vi "FRC Particle Classification Example.vi"() -> (1 "Highest Avg Score":dbl)   [LabVIEW 2015]
uses:
  <vilib>/Rock Robotics/WPI/Camera/WPI_CameraSettings Read MJPG.ctl
  <vilib>/Rock Robotics/WPI/Camera/WPI_CameraImageSize.ctl
  D:/LabView 2015/examples/FRC/roboRIO/Vision/2016 Vision Example/Vision Support Code/Camera Types.ctl
  <vilib>/vision/NI_Vision_Development_Module.lvlib
panel:
  in  "Std Devs for Calibration":cluster{"H":dbl, "S":dbl, "V":dbl}={"H"=4.0, "S"=6.0, "V"=6.0}
  in  "Min Score Threshold":i32=70
  in  "Camera Type":T1=enum."MS HD3000 square"
  in  "image files":string[](array[string])
  out "Detected Targets":T2(array[cluster]) {"Normalized Rect"."Numeric 5" format="%#_2g"; "Normalized Rect"."Numeric 3" format="%#_2g"; "Normalized Rect"."Numeric 2" format="%#_2g"; "Normalized Rect"."Numeric" format="%#_2g"}
  in  "Annotation Limit":dbl=75.0
  in  "Source":enum32{"Files", "Camera"}(tab)
  in  "Images":i32(listbox)
  in  "Folder Location":path=path "C:/Program Files (x86)/National Instruments/LabVIEW 2015/examples/FRC/roboRIO/Vision/2016 Vision Example/Sample Images/Real Tower"
  in  "Camera Settings":T3={"fps"=20, "compression"=30, "Image Size"=enum."320x240"}
  in  "Camera Address":string="USB 1"
  in  "Annotate":bool=TRUE
  out "Sorted Scores":T5(array[cluster]) {"?" format="%#_3g"; "Class Score" format="%#_3g"}
  out "Qualified Particles":i32
  in  "LED Color":T6={"Hue"={110.68604567358754, 149.18771039657545}, "Sat"={35.35714285714287, 255.0}, "Val"={91.0, 255.0}} {"Hue" scale=0.0..255.0 scale format="%#_3g"}
  out "Masked":T7(plugin-control)
  out "Original Image":T7(plugin-control)
  # "Instructions:\nUse Source to select image files from a directory, or use a USB or IP camera connected to your laptop.\nUse LED Color to threshold and build particles. Adjust HSV values to improve masking.\nClick and draw a line in Original Image to auto-calibrate to the LED color. You may need to widen Sat and Val.\nAnnotations draw a rectangle around \"good\" particles with scores from top to bottom."
  # "ID Score"
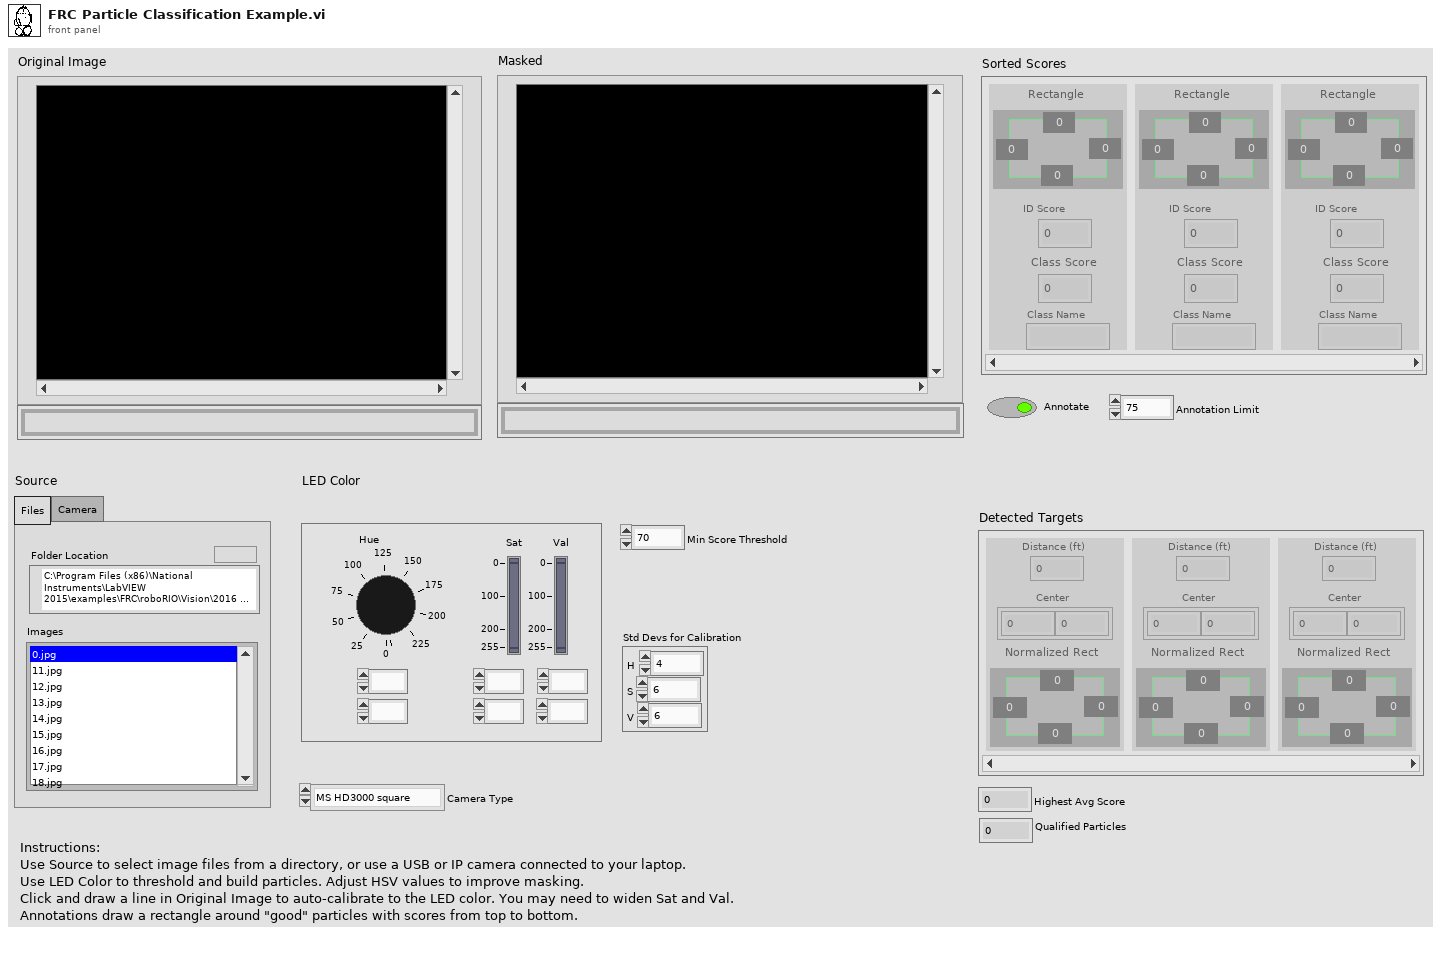
[diagram p1: front panel]
types:
  T1 = typedef "Camera Types.ctl" = enum16{"206", "1011", "1013", "MS HD3000 square", "MS HD3000 640x480"}
  T2 = cluster{"Distance (ft)":dbl, "Center":cluster{dbl, dbl}, "Normalized Rect":cluster{"Numeric":dbl, "Numeric 2":dbl, "Numeric 3":dbl, "Numeric 5":dbl}}[]
  T3 = typedef "WPI_CameraSettings Read MJPG.ctl" = cluster{"fps":i32, "compression":i32, "Image Size":T4}
  T4 = typedef "WPI_CameraImageSize.ctl" = enum16{"640x480", "320x240", "160x120", "Custom"}
  T5 = cluster{"Rectangle":cluster{"Numeric":dbl, "Numeric 2":dbl, "Numeric 3":dbl, "Numeric 5":dbl}, dbl, "Class Score":dbl, "Class Name":string}[]
  T6 = cluster{"Hue":cluster{dbl, dbl}, "Sat":cluster{dbl, dbl}, "Val":cluster{dbl, dbl}}
  T7 = typedef "IMAQ Image.ctl" = refnum<image>
  T8 = typedef "Particle Parameters" = i32
  T9 = typedef "Image Type" = u32
  T10 = typedef "IMAQ Classifier Session.ctl" = refnum<k1>
  T11 = cluster{"Numeric":dbl, "Numeric":dbl, "Numeric":dbl, "Numeric":dbl, dbl}
  T12 = cluster{cluster{dbl, dbl}, cluster{dbl, dbl}, cluster{dbl, dbl}}
  T13 = typedef "ROI Descriptor" = cluster{"Global Rectangle":i32[], "Contours":cluster{"ID":enum32{"External", "Internal"}, "Type":u32, "Coordinates":i32[]}[]}
  T14 = cluster{"Classification Score":sgl, "Identification Score":sgl}
  T15 = cluster{"Classification Score":dbl, "Identification Score":dbl}
  T16 = cluster{"Numeric":dbl, "Numeric":dbl, "Numeric":dbl, "Numeric":dbl}
  T17 = cluster{cluster{"Numeric":dbl, "Numeric":dbl, "Numeric":dbl, "Numeric":dbl}, "Identification Score":dbl, "Classification Score":dbl, "Class":string}
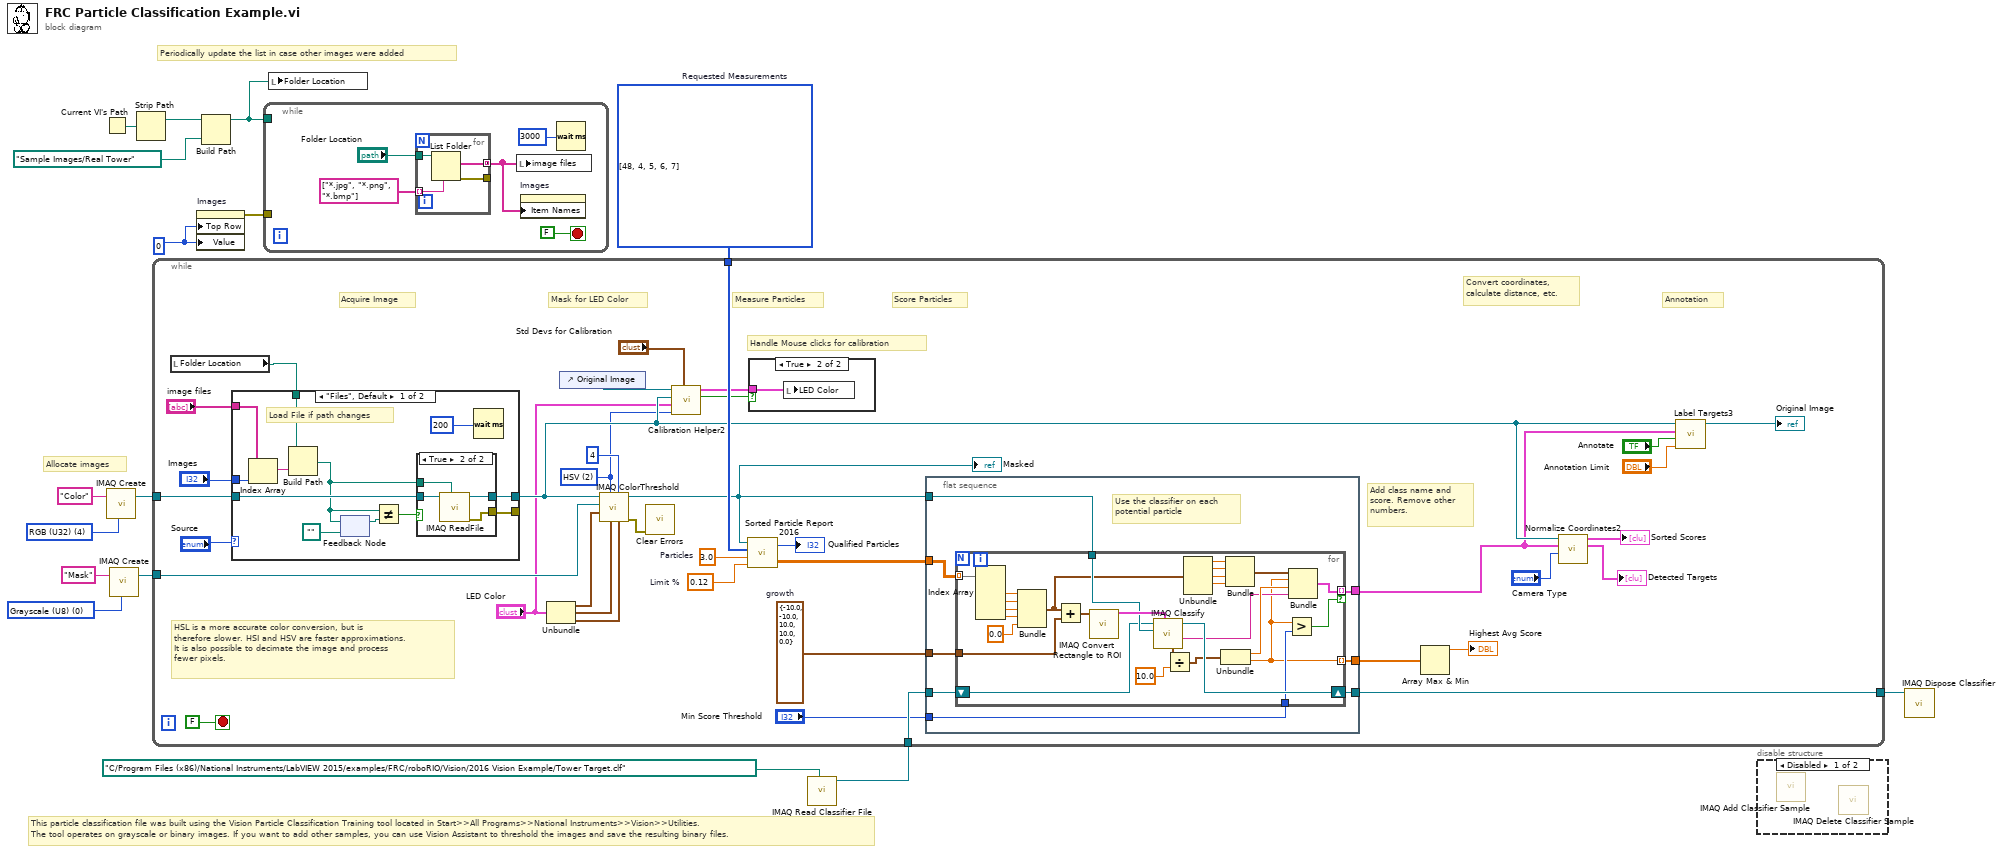
[diagram p0: block diagram]
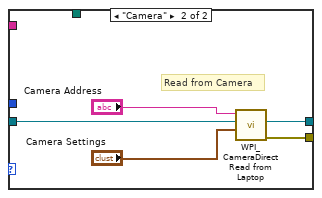
[diagram p5: hidden frame]
diagram:
  w3 = u32 0 ("milliseconds to wait")
  w10 = T8[] [48, 4, 5, 6, 7] items=["Center of Mass X", "Center of Mass Y", "First Pixel X", "First Pixel Y", "Bounding Rect Left", "Bounding Rect Top", "Bounding Rect Right", "Bounding Rect Bottom", "Max Feret Diameter Start X", "Max Feret Diameter Start Y", "Max Feret Diameter End X", "Max Feret Diameter End Y", "Max Horiz. Segment Length Left", "Max Horiz. Segment Length Right", "Max Horiz. Segment Length Row", "-", "Bounding Rect Width", "Bounding Rect Height", "Bounding Rect Diagonal", "Perimeter", "Convex Hull Perimeter", "Holes' Perimeter", "Max Feret Diameter", "Equivalent Ellipse Major Axis", "Equivalent Ellipse Minor Axis", "Equivalent Ellipse Minor Axis (Feret)", "Equivalent Rect Long Side", "Equivalent Rect Short Side", "Equivalent Rect Diagonal", "Equivalent Rect Short Side (Feret)", "Average Horiz. Segment Length", "Average Vert. Segment Length", "Hydraulic Radius", "Waddel Disk Diameter", "-", "Area", "Holes' Area", "Particle & Holes' Area", "Convex Hull Area", "Image Area", "-", "Number of Holes", "Number of Horiz. Segments", "Number of Vert. Segments", "-", "Orientation", "Max Feret Diameter Orientation", "-", "% Area/Image Area", "% Area/(Particle & Holes' Area)", "Ratio of Equivalent Ellipse Axes", "Ratio of Equivalent Rect Sides", "-", "Elongation Factor", "Compactness Factor", "Heywood Circularity Factor", "Type Factor", "-", "Sum X", "Sum Y", "Sum XX", "Sum XY", "Sum YY", "Sum XXX", "Sum XXY", "Sum XYY", "Sum YYY", "-", "Moment of Inertia XX", "Moment of Inertia XY", "Moment of Inertia YY", "Moment of Inertia XXX", "Moment of Inertia XXY", "Moment of Inertia XYY", "Moment of Inertia YYY", "Norm. Moment of Inertia XX", "Norm. Moment of Inertia XY", "Norm. Moment of Inertia YY", "Norm. Moment of Inertia XXX", "Norm. Moment of Inertia XXY", "Norm. Moment of Inertia XYY", "Norm. Moment of Inertia YYY", "Hu Moment 1", "Hu Moment 2", "Hu Moment 3", "Hu Moment 4", "Hu Moment 5", "Hu Moment 6", "Hu Moment 7"]  # Requested Measurements
  w13 = T9 0 items=["Grayscale (U8)", "Grayscale (I16)", "Grayscale (SGL)", "Complex (CSG)", "RGB (U32)", "HSL (U32)", "RGB (U64)", "Grayscale (U16)"] ("Image Type")
  w15 = T9 4 items=["Grayscale (U8)", "Grayscale (I16)", "Grayscale (SGL)", "Complex (CSG)", "RGB (U32)", "HSL (U32)", "RGB (U64)", "Grayscale (U16)"] ("Image Type")
  # "This particle classification file was built using the Vision Particle Classification Training tool located in Start>>All Programs>>National Instruments>>Vision>>Utilities.\nThe tool operates on grayscale or binary images. If you want to add other samples, you can use Vision Assistant to threshold the images and save the resulting binary files."
  # "Periodically update the list in case other images were added"
  # "Allocate images"
  n1 = Current VI's Path() -> (path=w9:path)
  n2 = call "IMAQ Create"("Image Name"="Color", "Image Type"=w15) -> ("New Image"=w14:T7)  [unwired: 2 in, 2 out]
  n3 = call "IMAQ Create"("Image Name"="Mask", "Image Type"=w13) -> ("New Image"=w11:T7)  [unwired: 2 in, 2 out]
  n4 = Strip Path(path=w9) -> (stripped path=w4:path)  [unwired: 1 out]
  n5 = property on="Images" class="LstBox (strict)"("Top Row"=w3, "Value"=w3) -> (error out=w2:errorcluster)  [unwired: 2 in, 1 out]
  n6 = Build Path(base path=w4, name or relative path=path "Sample Images/Real Tower" ("Folder Location")) -> (appended path=w1:path)
  n7 = while {
    tunnel: w1 -> [_]
    tunnel: w2 -> [_]
    stop <- FALSE stop-if-true
    n8 = for {
      tunnel: [w25] -> w19 mode=concatenating
      tunnel: "Folder Location" -> [w24]
      tunnel: [w23] -> _
      tunnel: string[] ["*.jpg", "*.png", "*.bmp"] -> [w22] mode=indexing
      n9 = List Folder(path=w24, pattern=w22) -> (filenames=w25:string[], error out=w23:errorcluster)  [unwired: 2 in, 2 out]
    }
    n10 = local write "image files"(w19) -> ()
    n11 = property on="Images" class="LstBox (strict)"("Item Names"=w19) -> ()  [unwired: 2 in, 2 out]
    n12 = Wait (ms)(milliseconds to wait=u32 3000) -> ()  [unwired: 1 out]
  }
  n13 = local write "Folder Location"(w1) -> ()
  n14 = call "IMAQ Read Classifier File"("File Path"=path "C:/Program Files (x86)/National Instruments/LabVIEW 2015/examples/FRC/roboRIO/Vision/2016 Vision Example/Tower Target.clf" ("appended path")) -> ("Classifier Session"=w7:T10)  [unwired: 3 in, 7 out]
  n15 = while {
    tunnel: w14 -> [w62]
    tunnel: w11 -> [w60]
    tunnel: w10 -> [w56]
    tunnel: w7 -> [w38]
    tunnel: [w35] -> w6
    stop <- FALSE stop-if-true
    w39 = T11 {"Numeric"=-10.0, "Numeric"=-10.0, "Numeric"=10.0, "Numeric"=10.0, 0.0}  # growth
    w53 = 0.12  # Limit %
    w55 = 3.0  # Particles
    w43 = u16 2 items=["RGB", "HSL", "HSV", "HSI"] ("Color Mode")
    # "Add class name and\nscore. Remove other\nnumbers."
    # "Handle Mouse clicks for calibration"
    # "Measure Particles"
    # "Convert coordinates,\ncalculate distance, etc."
    # "Annotation"
    # "Score Particles"
    # "Mask for LED Color"
    # "Acquire Image"
    # "HSL is a more accurate color conversion, but is\ntherefore slower. HSI and HSV are faster approximations.\nIt is also possible to decimate the image and process\nfewer pixels."
    n16 = local read "Folder Location"() -> (w26:path)
    n17 = case shown="\"Files\", Default" "Source" {
      tunnel: [w110 w121] -> _
      tunnel: [w111 w120] -> w46
      tunnel: w62 -> [w109 w119]
      tunnel: "image files" -> [w101 _]
      tunnel: "Images" -> [w108 _]
      tunnel: w26 -> [w106 _]
      frame "Files", Default {
        # "Load File if path changes"
        n18 = Index Array(array=w101, index=w108) -> (element=w107:string)
        n19 = Build Path(base path=w106, name or relative path=w107) -> (appended path=w102:path)
        n20 = feedback-in #1(w102) -> ()
        n21 = feedback #1(path "" ("appended path")) -> (w104:path)
        n22 = Not Equal?(x=w102, y=w104) -> (x != y?=w105:bool)
        n23 = case shown="True" w105 {
          tunnel: [w112 w116] -> w111
          tunnel: [_ w115] -> w110
          tunnel: w109 -> [w112 w114]
          tunnel: w102 -> [_ w113]
          frame False {
          }
          frame True {
            n24 = call "IMAQ ReadFile"("File Path"=w113, "Image"=w114) -> ("error out"=w115:errorcluster, "Image Out"=w116:T7)  [unwired: 5 in, 3 out]
          }
        }
        n25 = Wait (ms)(milliseconds to wait=u32 200 ("delay (ms)")) -> ()  [unwired: 1 out]
      }
      frame "Camera" {
        # "Read from Camera"
        n26 = call <vilib>:"WPI_CameraDirect Read from Laptop.vi"("Camera Settings"="Camera Settings", "Image"=w119, "address"="Camera Address") -> ("error out"=w121:errorcluster, "Image Out"=w120:T7)  [unwired: 7 in]
      }
    }
    n27 = Unbundle("LED Color") -> ("Hue"=w59:cluster{dbl, dbl}, "Sat"=w58:cluster{dbl, dbl}, "Val"=w57:cluster{dbl, dbl})
    n28 = control-ref of="Original Image"() -> (w47:refnum<vi>)
    n29 = call "IMAQ ColorThreshold"("Blue or Luma or Val or Inten Range"=w57, "Replace Value"=4, "Green or Sat Range"=w58, "Color Mode"=w43, "Red or Hue Range"=w59, "Image Dst"=w60, "Image Src"=w46) -> ("error out"=w48:errorcluster, "Image Dst Out"=w37:T7)  [unwired: 3 in]
    "Masked" <- w37
    n30 = call <vilib>:"Clear Errors.vi"("error in (no error)"=w48) -> ()  [unwired: 5 in, 2 out]
    n31 = call "Calibration Helper2.vi"("Std Devs"="Std Devs for Calibration", "Color Mode"=w43, "Color Components"="LED Color", "Image"=w46, "Image Ctl Refnum"=w47) -> ("Changed"=w45:bool, "output color"=w44:T12)  [unwired: 5 in]
    n32 = call "Sorted Particle Report 2016.vi"("Min Area Size %"=w53, "Particle Count Limit"=w55, "Pixel Measurements"=w56, "Image in"=w37) -> ("Sorted Data"=w40:dbl[][], "Particles"=→"Qualified Particles":i32)
    n33 = case shown="True" w45 {
      tunnel: w44 -> [_ w64]
      frame False {
      }
      frame True {
        n34 = local write "LED Color"(w64) -> ()
      }
    }
    n35 = flat-sequence {
      tunnel: w38 -> [w69]
      tunnel: [w67] -> w29
      tunnel: [w66] -> w35
      tunnel: [w65] -> w27
      tunnel: w40 -> [w72]
      tunnel: w39 -> [w71]
      tunnel: w37 -> [w70]
      tunnel: "Min Score Threshold" -> [w68]
      frame #0 {
        # "Use the classifier on each\npotential particle"
        n36 = for {
          tunnel: w72 -> [w99] mode=indexing
          tunnel: w68 -> [w87]
          tunnel: w71 -> [w92]
          tunnel: w70 -> [w90]
          shift-right: [w88] -> w66
          shift-left: w69 -> [w89]
          tunnel: [w76] -> w65 mode=indexing
          tunnel: [w85] -> w67 mode=indexing if=w86
          n37 = Index Array(array=w99) -> (element #2=w97:dbl, element #3=w96:dbl, element #4=w94:dbl, element #5=w95:dbl)  [unwired: 5 in, 1 out]
          n38 = Bundle("Numeric"=w97, "Numeric"=w96, "Numeric"=w94, "Numeric"=w95, 0.0) -> (w84:T11)  [unwired: 1 out]
          n39 = Add(x=w84, y=w92) -> (x+y=w93:T11)
          n40 = call "IMAQ Convert Rectangle to ROI"("Rectangle"=w93) -> ("ROI Descriptor"=w91:T13)  [unwired: 1 in, 8 out]
          n41 = call "IMAQ Classify"("ROI Descriptor"=w91, "Image"=w90, "Classifier Session"=w89) -> ("Class"=w77:string, "Classifier Session (dup)"=w88:T10, "Scores"=w74:T14)  [unwired: 1 in, 5 out]
          n42 = Divide(x=w74, y=10.0) -> (x/y=w73:T15)
          n43 = Unbundle(w84) -> ("Numeric"=w82:dbl, "Numeric"=w81:dbl, "Numeric"=w80:dbl, "Numeric"=w79:dbl)  [unwired: 1 out]
          n44 = Unbundle(w73) -> ("Classification Score"=w78:dbl, "Identification Score"=w76:dbl)
          n45 = Bundle("Numeric"=w82, "Numeric"=w81, "Numeric"=w80, "Numeric"=w79) -> (w83:T16)  [unwired: 1 out]
          n46 = Greater?(x=w76, y=w87) -> (0:w86:bool)
          n47 = Bundle(w83, "Identification Score"=w76, "Classification Score"=w78, "Class"=w77) -> (w85:T17)  [unwired: 1 out]
        }
      }
    }
    n48 = Array Max & Min(array=w27) -> (max value=→"Highest Avg Score":dbl)  [unwired: 3 out]
    n49 = call "Normalize Coordinates2.vi"("Camera Type"="Camera Type", "Targets"=w29, "Image in"=w46) -> ("Found Targets"=→"Detected Targets":T2, "Sorted Scores"=→"Sorted Scores":T5)  [unwired: 7 in]
    n50 = call "Label Targets3.vi"("Score Threshold"="Annotation Limit", "Annotate"="Annotate", "Targets"=w29, "Image in"=w46) -> ("Image out"=→"Original Image":T7)  [unwired: 7 in]
  }
  n51 = disable-structure shown="Disabled" {
    frame Disabled {
      n52 = call "IMAQ Add Classifier Sample"() -> ()  [unwired: 9 in, 3 out]
      n53 = call "IMAQ Delete Classifier Sample"() -> ()  [unwired: 10 in, 2 out]
    }
    frame Enabled {
    }
  }
  n54 = call "IMAQ Dispose Classifier"("Classifier Session"=w6) -> ()  [unwired: 1 in, 10 out]
